vi "build menu.vi"(8 "error in (no error)":errorcluster, 11 "UI elements cluster":T1) -> (0 "error out":errorcluster, 3 "UI elements cluster":T1)   [LabVIEW 2013]
uses:
  Typedefs/UI ctrl refs cluster.ctl
  Typedefs/Laser control knob.ctl
  Typedefs/Frame Size.ctl
  Typedefs/Plane Mode.ctl
  Typedefs/PMT control knob.ctl
  <vilib>/Utility/miscctls.llb/LVMenuShortCut.ctl
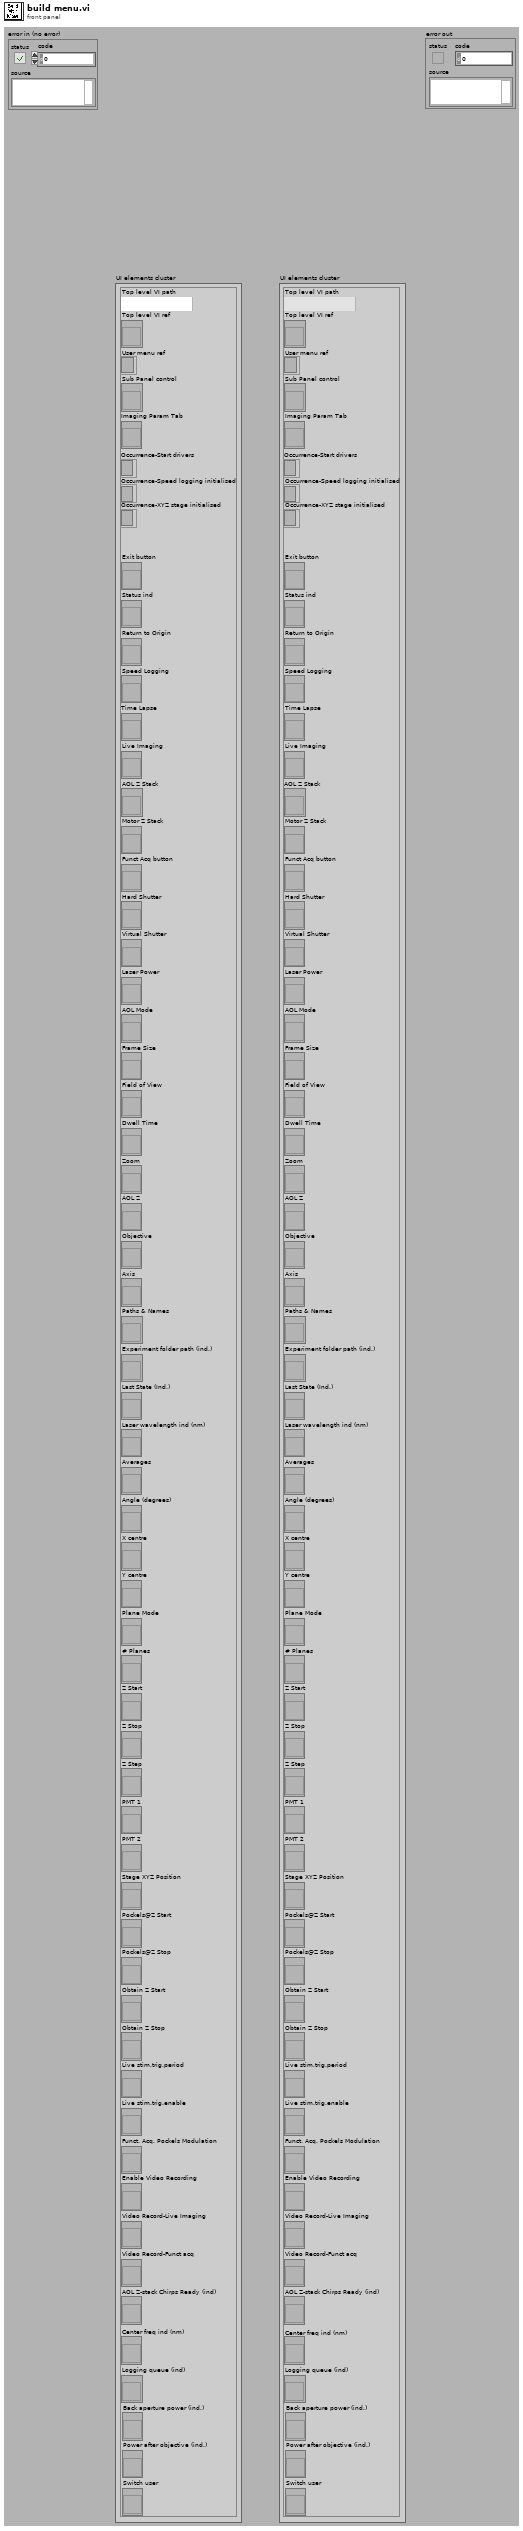
[diagram p1: front panel]
types:
  T1 = typedef "UI ctrl refs cluster.ctl" = cluster{"Top level VI path":path, "Top level VI ref":refnum<vi>, "User menu ref":refnum<k9>, "Sub Panel control":refnum<vi>, "Imaging Param Tab":refnum<vi>, "Occurrence-Start drivers":refnum<k4>, "Occurrence-Speed logging initialised":refnum<k4>, "Occurrence-XYZ stage initialised":refnum<k4>, "Exit button":refnum<vi>, "Status ind":refnum<vi>, "Return to Origin":refnum<vi>, "Speed Logging":refnum<vi>, "Time Lapse":refnum<vi>, "Live Imaging":refnum<vi>, "AOL Z Stack":refnum<vi>, "Motor Z Stack":refnum<vi>, "Funct Acq button":refnum<vi>, "Hard Shutter":refnum<vi>, "Virtual Shutter":refnum<vi>, "Laser Power":refnum<vi>, "AOL Mode":refnum<vi>, "Frame Size":refnum<vi>, "Field of View":refnum<vi>, "Dwell Time":refnum<vi>, "Zoom":refnum<vi>, "AOL Z":refnum<vi>, "Objective":refnum<vi>, "Axis":refnum<vi>, "Paths & Names":refnum<vi>, "Experiment folder path (ind.)":refnum<vi>, "Last State (Ind.)":refnum<vi>, "Laser wavelength ind (nm)":refnum<vi>, "Averages":refnum<vi>, "Angle (degrees)":refnum<vi>, "X centre":refnum<vi>, "Y centre":refnum<vi>, "Plane Mode":refnum<vi>, "# Planes":refnum<vi>, "Z Start":refnum<vi>, "Z Stop":refnum<vi>, "Z Step":refnum<vi>, "PMT 1":refnum<vi>, "PMT 2":refnum<vi>, "Stage XYZ Position":refnum<vi>, "Pockels@Z Start":refnum<vi>, "Pockels@Z Stop":refnum<vi>, "Obtain Z Start":refnum<vi>, "Obtain Z Stop":refnum<vi>, "Live stim.trig.period":refnum<vi>, "Live stim.trig.enable":refnum<vi>, "Funct. Acq. Pockels Modulation":refnum<vi>, "Enable Video Recording":refnum<vi>, "Video Record-Live Imaging":refnum<vi>, "Video Record-Funct acq":refnum<vi>, "AOL Z-stack Chirps Ready (ind)":refnum<vi>, "Center freq ind (nm)":refnum<vi>, "Logging queue (ind)":refnum<vi>, "Back aperture power (ind.)":refnum<vi>, "Power after objective (ind.)":refnum<vi>, "Switch user":refnum<vi>}
  T2 = typedef "LVMenuShortCut.ctl" = cluster{"Include Shift Key?":bool, "Include Ctrl Key?":bool, "Shortcut Key":string}
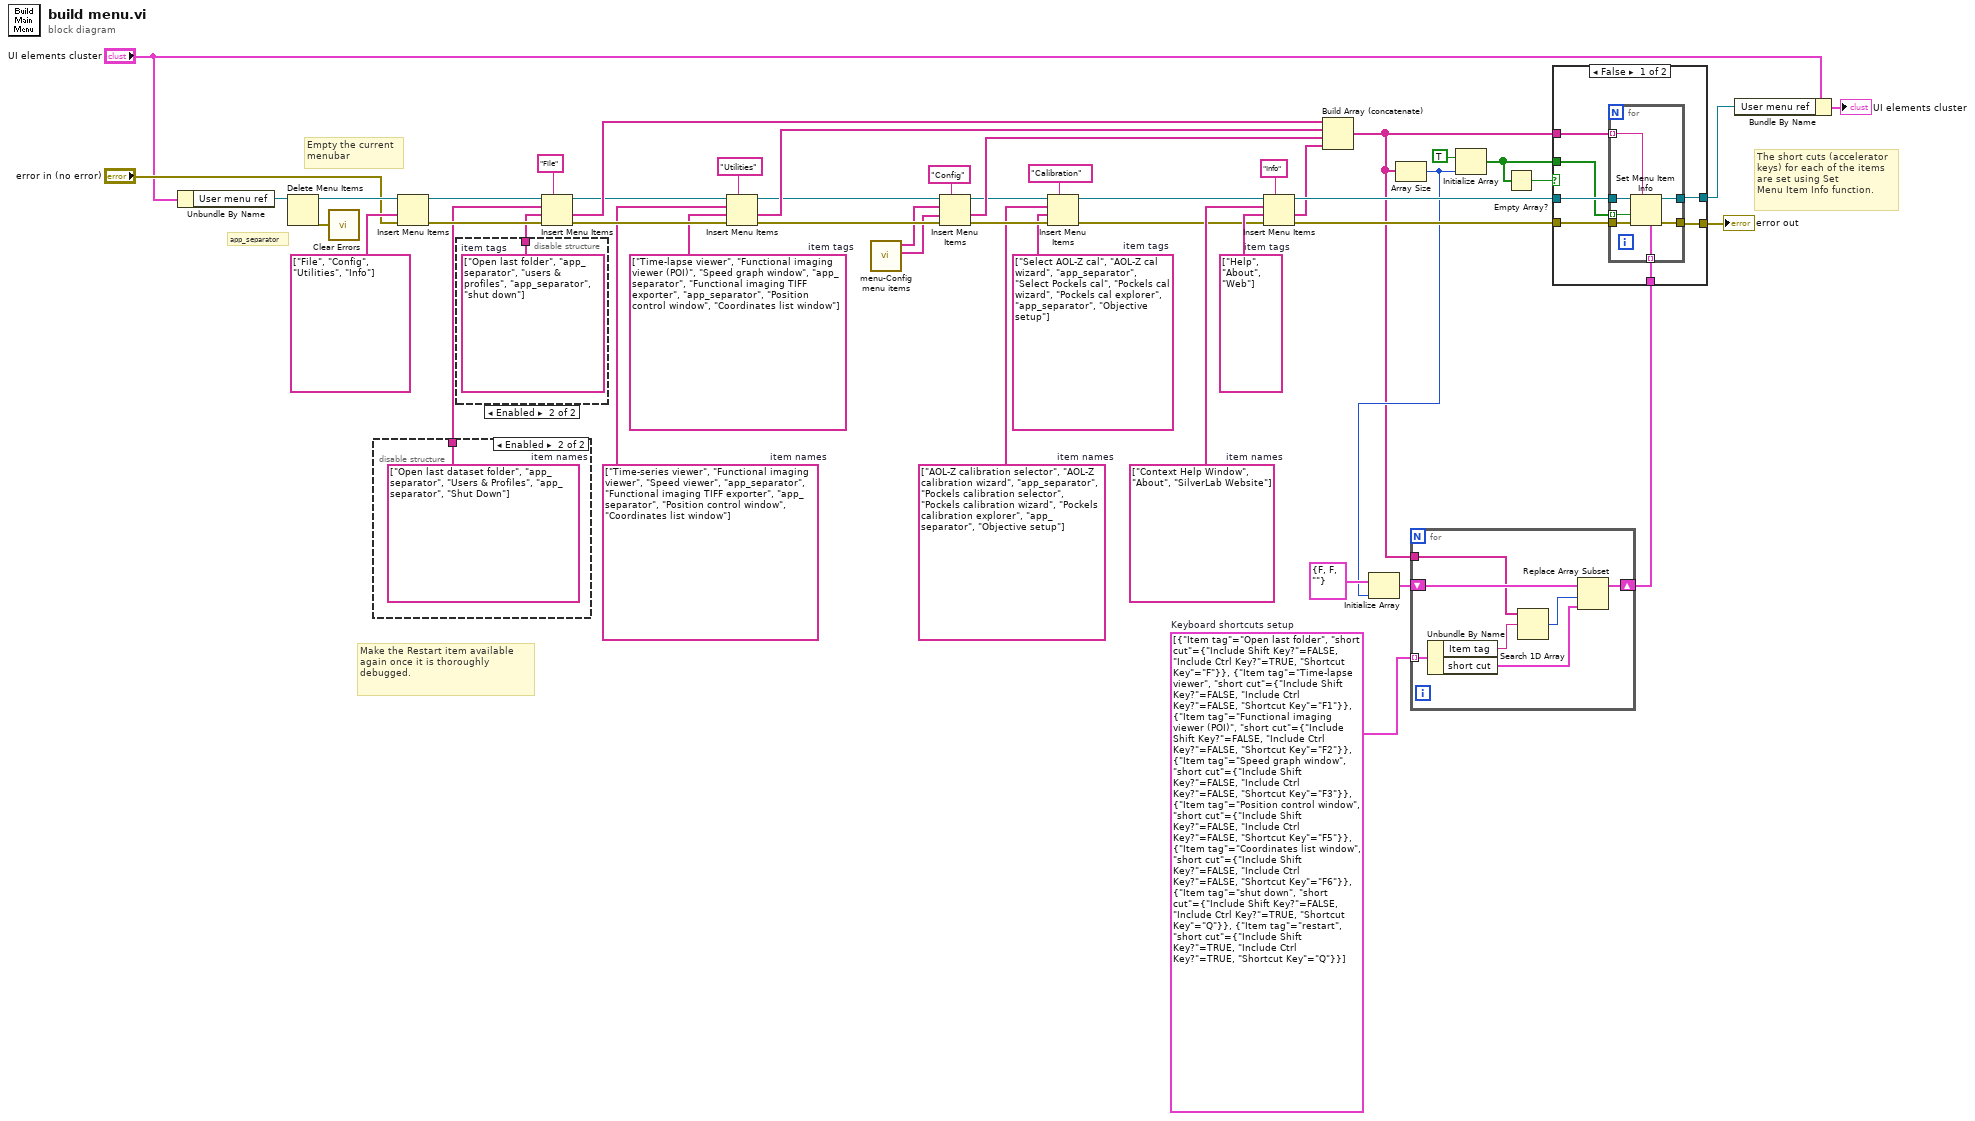
[diagram p0: block diagram]
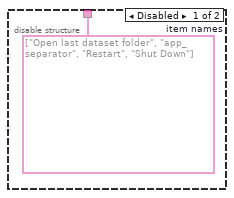
[diagram p3: hidden frame]
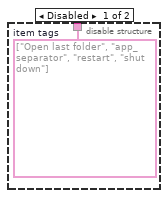
[diagram p4: hidden frame]
diagram:
  w9 = cluster{"Item tag":string, "short cut":T2}[] [{"Item tag"="Open last folder", "short cut"={"Include Shift Key?"=FALSE, "Include Ctrl Key?"=TRUE, "Shortcut Key"="F"}}, {"Item tag"="Time-lapse viewer", "short cut"={"Include Shift Key?"=FALSE, "Include Ctrl Key?"=FALSE, "Shortcut Key"="F1"}}, {"Item tag"="Functional imaging viewer (POI)", "short cut"={"Include Shift Key?"=FALSE, "Include Ctrl Key?"=FALSE, "Shortcut Key"="F2"}}, {"Item tag"="Speed graph window", "short cut"={"Include Shift Key?"=FALSE, "Include Ctrl Key?"=FALSE, "Shortcut Key"="F3"}}, {"Item tag"="Position control window", "short cut"={"Include Shift Key?"=FALSE, "Include Ctrl Key?"=FALSE, "Shortcut Key"="F5"}}, {"Item tag"="Coordinates list window", "short cut"={"Include Shift Key?"=FALSE, "Include Ctrl Key?"=FALSE, "Shortcut Key"="F6"}}, {"Item tag"="shut down", "short cut"={"Include Shift Key?"=FALSE, "Include Ctrl Key?"=TRUE, "Shortcut Key"="Q"}}, {"Item tag"="restart", "short cut"={"Include Shift Key?"=TRUE, "Include Ctrl Key?"=TRUE, "Shortcut Key"="Q"}}]  # Keyboard shortcuts setup
  w15 = string[] ["AOL-Z calibration selector", "AOL-Z calibration wizard", "app_separator", "Pockels calibration selector", "Pockels calibration wizard", "Pockels calibration explorer", "app_separator", "Objective setup"]  # item names
  w19 = string[] ["Time-series viewer", "Functional imaging viewer", "Speed viewer", "app_separator", "Functional imaging TIFF exporter", "app_separator", "Position control window", "Coordinates list window"]  # item names
  w21 = string[] ["Select AOL-Z cal", "AOL-Z cal wizard", "app_separator", "Select Pockels cal", "Pockels cal wizard", "Pockels cal explorer", "app_separator", "Objective setup"]  # item tags
  w20 = string[] ["Time-lapse viewer", "Functional imaging viewer (POI)", "Speed graph window", "app_separator", "Functional imaging TIFF exporter", "app_separator", "Position control window", "Coordinates list window"]  # item tags
  w30 = string[] ["Context Help Window", "About", "SilverLab Website"]  # item names
  w32 = string[] ["Help", "About", "Web"]  # item tags
  # "Make the Restart item available again once it is thoroughly debugged."
  # "app_separator"
  # "Empty the current\nmenubar"
  # "The short cuts (accelerator\nkeys) for each of the items\nare set using Set\nMenu Item Info function."
  n1 = Unbundle By Name("UI elements cluster") -> ("User menu ref"=w6:refnum<k9>)
  n2 = Delete Menu Items(9:w6) -> (0:w38:errorcluster, 3:w45:refnum<k9>)  [unwired: 2 in, 1 out]
  n3 = call <vilib>:"Clear Errors.vi"("error in (no error)"=w38) -> ()  [unwired: 6 in, 1 out]
  n4 = disable-structure shown="Enabled" {
    disable-tunnel: [w50 w51] -> w16
    frame Disabled {
      w50 = string[] ["Open last dataset folder", "app_separator", "Restart", "Shut Down"]  # item names
    }
    frame Enabled {
      w51 = string[] ["Open last dataset folder", "app_separator", "Users & Profiles", "app_separator", "Shut Down"]  # item names
    }
  }
  n5 = Insert Menu Items(6:"error in (no error)", 7:string[] ["File", "Config", "Utilities", "Info"] ("item tags"), 9:w45) -> (0:w46:errorcluster, 3:w39:refnum<k9>)  [unwired: 4 out]
  n6 = disable-structure shown="Enabled" {
    disable-tunnel: [w52 w53] -> w43
    frame Disabled {
      w52 = string[] ["Open last folder", "app_separator", "restart", "shut down"]  # item tags
    }
    frame Enabled {
      w53 = string[] ["Open last folder", "app_separator", "users & profiles", "app_separator", "shut down"]  # item tags
    }
  }
  n7 = Insert Menu Items(5:"File" ("menu tag"), 6:w46, 7:w43, 8:w16, 9:w39) -> (0:w47:errorcluster, 1:w44:string[], 3:w40:refnum<k9>)  [unwired: 1 out]
  n8 = Insert Menu Items(5:"Utilities" ("menu tag"), 6:w47, 7:w20, 8:w19, 9:w40) -> (0:w17:errorcluster, 1:w35:string[], 3:w18:refnum<k9>)  [unwired: 1 out]
  n9 = call "menu-Config menu items.vi"() -> ("item tags"=w7:string[], "item names"=w8:string[])  [unwired: 10 in]
  n10 = Insert Menu Items(5:"Config", 6:w17, 7:w7, 8:w8, 9:w18) -> (0:w25:errorcluster, 1:w33:string[], 3:w26:refnum<k9>)  [unwired: 1 out]
  n11 = Insert Menu Items(5:"Calibration", 6:w25, 7:w21, 8:w15, 9:w26) -> (0:w24:errorcluster, 3:w23:refnum<k9>)  [unwired: 2 out]
  n12 = Insert Menu Items(5:"Info" ("menu tag"), 6:w24, 7:w32, 8:w30, 9:w23) -> (0:w48:errorcluster, 1:w31:string[], 3:w42:refnum<k9>)  [unwired: 1 out]
  n13 = Build Array (concatenate)(w44, w35, w33, w31) -> (w10:string[])
  n14 = Array Size(array=w10) -> (size(s)=w11:i32)
  n15 = Initialize Array(T2 {"Include Shift Key?"=FALSE, "Include Ctrl Key?"=FALSE, "Shortcut Key"=""} ("short cut"), w11) -> (w12:T2[])
  n16 = for {
    shift-right: [w60] -> w13
    shift-left: w12 -> [w59]
    tunnel: w9 -> [w58] mode=indexing
    tunnel: w10 -> [w56]
    n17 = Unbundle By Name(w58) -> ("Item tag"=w55:string, "short cut"=w57:T2)
    n18 = Search 1D Array(1D array=w56, element=w55) -> (index of element=w54:i32)  [unwired: 1 in]
    n19 = Replace Array Subset(array=w59, new element=w57, index=w54) -> (w60:T2[])
  }
  n20 = Initialize Array(TRUE, w11) -> (w2:bool[])
  n21 = Empty Array?(array=w2) -> (empty?=w1:bool)
  n22 = case shown="False" w1 {
    tunnel: [w67 w75] -> w49
    tunnel: w48 -> [w66 w75]
    tunnel: w42 -> [w65 w76]
    tunnel: w13 -> [w64 _]
    tunnel: w10 -> [w63 _]
    tunnel: [w62 w76] -> w4
    tunnel: w2 -> [w61 _]
    frame False {
      n23 = for {
        tunnel: w65 -> [w74]
        tunnel: [w73] -> w62
        tunnel: w63 -> [w72] mode=indexing
        tunnel: w66 -> [w71]
        tunnel: [w70] -> w67
        tunnel: w61 -> [w69] mode=indexing
        tunnel: w64 -> [w68] mode=indexing
        n24 = Set Menu Item Info(4:w68, 7:w72, 8:w71, 9:w69, 11:w74) -> (0:w70:errorcluster, 3:w73:refnum<k9>)  [unwired: 2 out]
      }
    }
    frame True {
      # "Fail-safe case"
    }
  }
  "error out" <- w49
  n25 = Bundle By Name(cluster="UI elements cluster", "User menu ref"=w4) -> (→"UI elements cluster":T1)
